vi "Insert Value (Value[]).vi"(7 "keys":string[](array[string]), 8 "error in (no error)":errorcluster, 10 "values":refnum<class "JSON Value.lvclass">[](array[class]), 11 "JSON Value in":refnum<class "JSON Value.lvclass">) -> (0 "error out":errorcluster, 1 "replaced?":bool[](array[boolean]), 3 "JSON Value out":refnum<class "JSON Value.lvclass">)   [LabVIEW 2016, in "JSON Value.lvclass"]
uses:
  JSON Value.lvclass
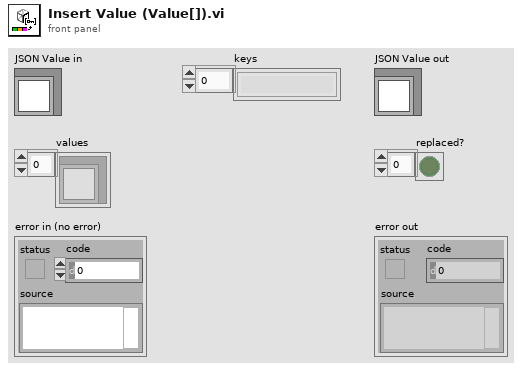
[diagram p1: front panel]
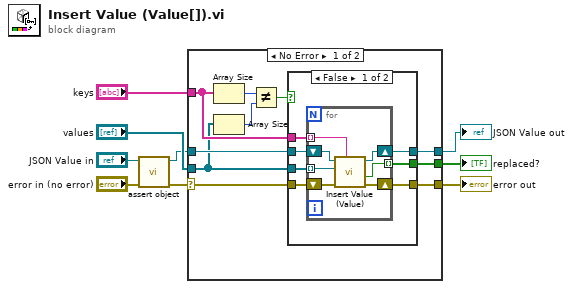
[diagram p0: block diagram]
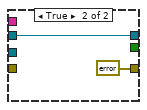
[diagram p2: hidden frame]
diagram:
  n1 = call "assert object.vi"("error in (no error)"="error in (no error)", "JSON Value in"="JSON Value in") -> ("error out"=w3:errorcluster, "JSON Value out"=w1:refnum<class "JSON Value.lvclass">)  [unwired: 8 in]
  n2 = case shown="No Error" w3 {
    selector: w3 -> [w16 w37]
    tunnel: [w15 w37] -> w8
    tunnel: [w13 w36] -> w7
    tunnel: w1 -> [w14 w36]
    tunnel: "keys" -> [w12 _]
    tunnel: "values" -> [w11 _]
    tunnel: [w10 _] -> w4
    frame No Error {
      n3 = Array Size(array=w12) -> (size(s)=w19:i32)
      n4 = Array Size(array=w11) -> (size(s)=w18:i32)
      n5 = Not Equal?(x=w19, y=w18) -> (x != y?=w17:bool)
      n6 = case shown="False" w17 {
        tunnel: w16 -> [w24 _]
        tunnel: [w23 errorcluster {"status"=TRUE, "code"=-1000, "source"="There must be an equal number of keys and values"} ("error constant")] -> w15
        tunnel: w14 -> [w26 w34]
        tunnel: [w25 w34] -> w13
        tunnel: w12 -> [w22 _]
        tunnel: w11 -> [w21 _]
        tunnel: [w20 _] -> w10
        frame False {
          n7 = for {
            shift-right: [w32] -> w25
            shift-left: w26 -> [w33]
            shift-right: [w30] -> w23
            shift-left: w24 -> [w31]
            tunnel: w22 -> [w29] mode=indexing
            tunnel: w21 -> [w28] mode=indexing
            tunnel: [w27] -> w20 mode=indexing
            n8 = call "Insert Value (Value).vi"("key"=w29, "error in (no error)"=w31, 10:"JSON Value in"=w28, 11:"JSON Value in"=w33) -> ("error out"=w30:errorcluster, "replaced"=w27:bool, "JSON Value out"=w32:refnum<class "JSON Value.lvclass">)  [unwired: 5 in]
          }
        }
        frame True {
        }
      }
    }
    frame Error {
    }
  }
  "error out" <- w8
  "JSON Value out" <- w7
  "replaced?" <- w4
